vi "SplittersTrialWindow.vi"() -> ()   [LabVIEW 2013]
panel:
  out "Live Absorption Spectrum":T1(graph)
  out "Live Spectrum":T1(graph)
  out "Dark Spectrum":T1(graph)
  out "Reference Spectrum":T1(graph)
  in  "Light Strobe Control":bool=TRUE
  in  "Number of\nsamples to average":i32=1 min=1 max=100 step=1
  in  "Take Ref Spectrum":bool
  in  "Take Dark Spectrum":bool
  out "Live samples for average":i32=1
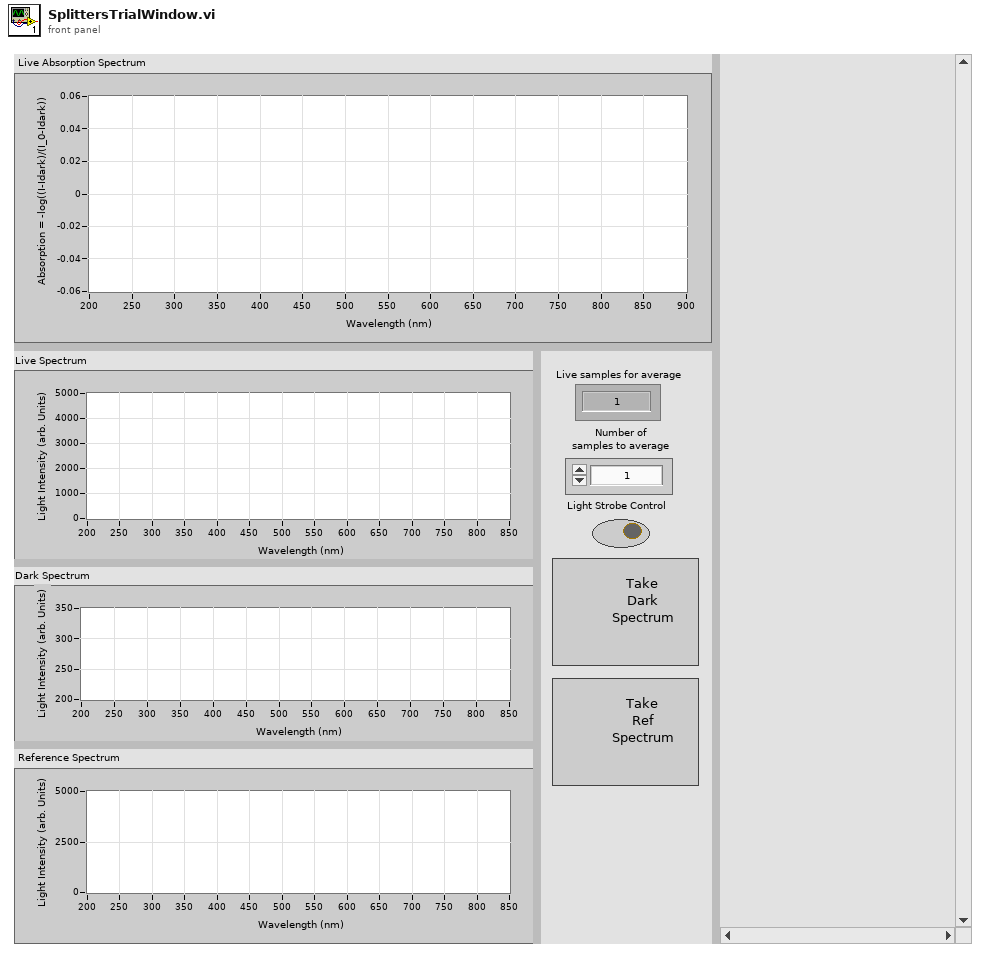
[diagram p1: front panel]
types:
  T1 = cluster{"Wavelength (nm)":dbl[], "Spectrum by Pixels":dbl[]}
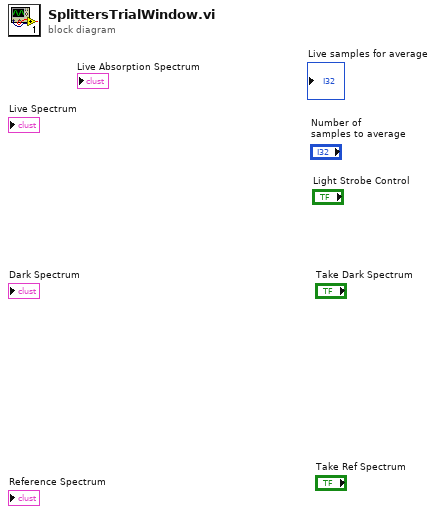
[diagram p0: block diagram]
diagram:
